vi "t0_from tf.vi"(5 "Open(t) Closed(f)":bool, 7 "Dt":dbl, 10 "Y":dbl[](array[numeric]), 11 "Tf":timestamp) -> (3 "New T0 Out":timestamp)   [LabVIEW 2024]
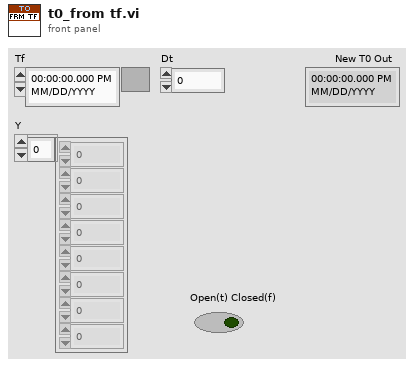
[diagram p1: front panel]
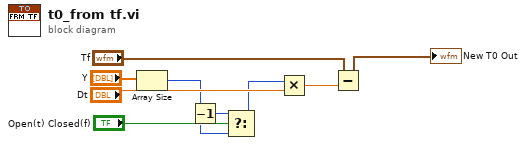
[diagram p0: block diagram]
diagram:
  n1 = Array Size(array="Y") -> (size(s)=w1:i32)
  n2 = Decrement(x=w1) -> (x-1=w2:i32)
  n3 = Select(t=w2, s="Open(t) Closed(f)", f=w1) -> (s? t:f=w3:i32)
  n4 = Multiply(x=w3, y="Dt") -> (x*y=w8:dbl)
  n5 = Subtract(x="Tf", y=w8) -> (x-y=→"New T0 Out":timestamp)
